vi "CommsTests.vi"() -> ()   [LabVIEW 2017]
uses:
  <vilib>/httpClient/LabVIEWHTTPClient.lvlib
panel:
  out "error out 2":errorcluster
  in  "remote port or service name":u16=2000
  in  "address":string="192.168.126.101"
  in  "data in":string="*SRHb\n"
  out "data out":string
  out "error out":errorcluster
  out "body":string
  out "headers":string="\r\n"
  in  "url":string="http://192.168.126.101"
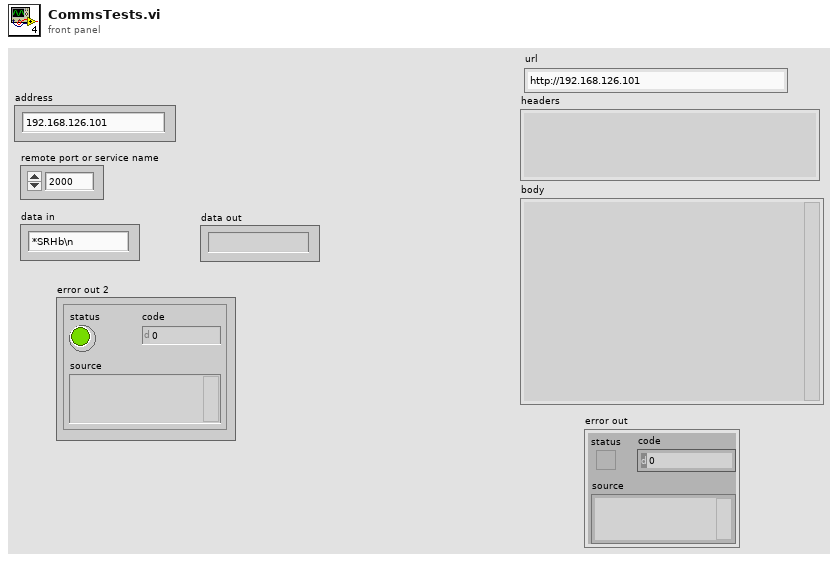
[diagram p1: front panel]
types:
  T1 = enum16{"Standard", "Buffered", "CRLF", "Immediate"}
  T2 = typedef "LabVIEWHTTPClient.lvlib/ClientHandle.ctl" = refnum<k1>
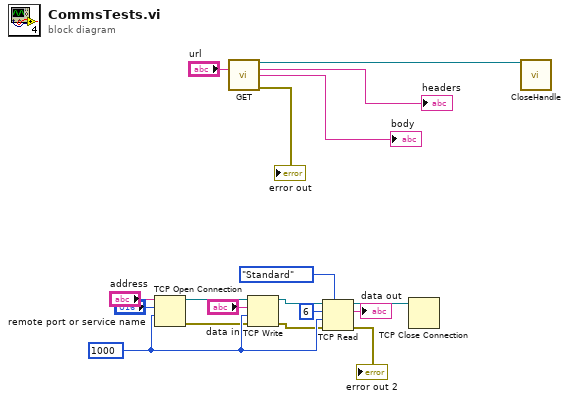
[diagram p0: block diagram]
diagram:
  w5 = 1000 ("timeout ms (60000)")
  n1 = TCP Open Connection(address="address", remote port or service name="remote port or service name", timeout ms (60000)=w5) -> (connection ID=w13:refnum<k5>, error out=w4:errorcluster)  [unwired: 2 in]
  n2 = call <vilib>:"GET.vi"("url"="url") -> ("client handle out"=w14:T2, "headers"=→"headers":string, "body"=→"body":string, "error out"=→"error out":errorcluster)  [unwired: 11 in]
  n3 = TCP Write(connection ID=w13, data in="data in", error in (no error)=w4, 9:w5) -> (connection ID out=w12:refnum<k5>, error out=w3:errorcluster)  [unwired: 1 out]
  n4 = TCP Read(connection ID=w12, bytes to read=6, error in (no error)=w3, 7:T1."Standard" ("mode (standard)"), 9:w5) -> (connection ID out=w11:refnum<k5>, data out=→"data out":string, error out=→"error out 2":errorcluster)
  n5 = TCP Close Connection(connection ID=w11) -> ()  [unwired: 2 in, 2 out]
  n6 = call <vilib>:"CloseHandle.vi"("client handle"=w14) -> ()  [unwired: 14 in, 1 out]
